vi "DMM Configuration - Update DMM Measurements ComboBox.vi"(8 "error in (no error)":errorcluster, 10 "Measurement":u16, 11 "Ring in":refnum<vi>) -> (0 "error out":errorcluster)   [LabVIEW 2015, in "DMM-SWITCH-ScanList System Explorer.lvlib"]
uses:
  DMM-SWITCH-ScanList System Explorer.lvlib
  Configuration Controls/DMM Config Function.ctl
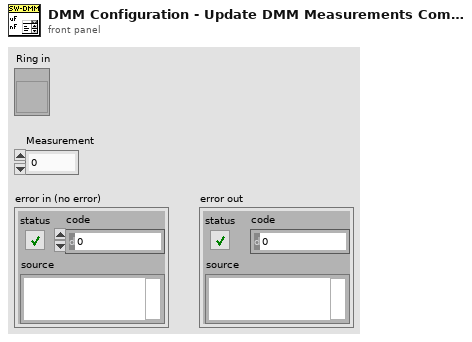
[diagram p1: front panel]
types:
  T1 = typedef "DMM-SWITCH-ScanList System Explorer.lvlib/DMM Config Function.ctl" = enum16{"DC Volts", "AC Volts", "DC Current", "AC Current", "2-wire Resistance", "4-wire Resistance", "Diode", "Frequency", "AC Volts DC Coupled", "Capacitance", "Inductance"}
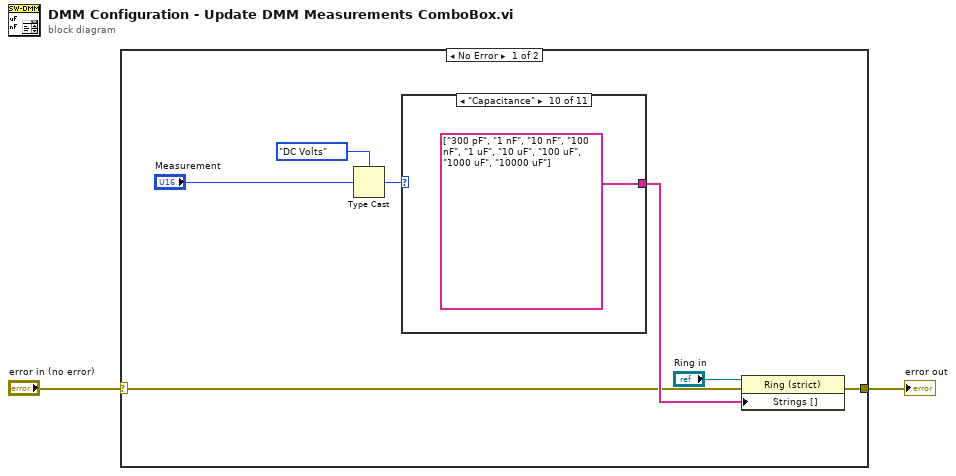
[diagram p0: block diagram]
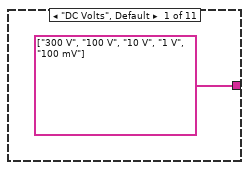
[diagram p2: hidden frame]
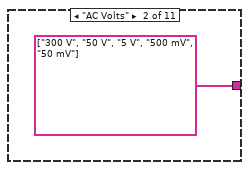
[diagram p3: hidden frame]
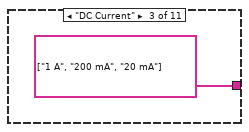
[diagram p4: hidden frame]
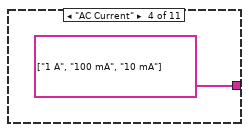
[diagram p5: hidden frame]
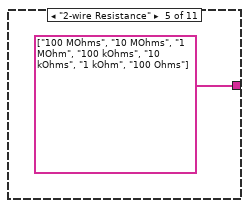
[diagram p6: hidden frame]
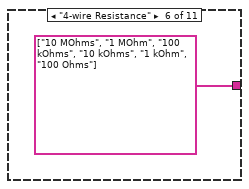
[diagram p7: hidden frame]
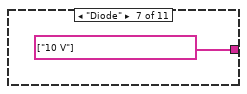
[diagram p8: hidden frame]
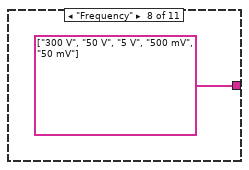
[diagram p9: hidden frame]
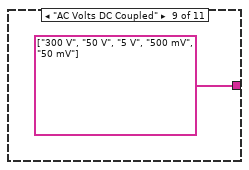
[diagram p10: hidden frame]
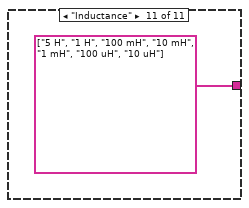
[diagram p11: hidden frame]
diagram:
  n1 = case shown="No Error" "error in (no error)" {
    selector: "error in (no error)" -> [w3 w21]
    tunnel: [w9 w21] -> w2
    frame No Error {
      n2 = Type Cast(type=DMM_Config_Function."DC Volts" ("Measurement Type Def"), x="Measurement") -> (*(type *) &x=w6:T1)
      n3 = case shown="\"Capacitance\"" w6 {
        tunnel: [string[] ["300 V", "100 V", "10 V", "1 V", "100 mV"] ("Strings []") string[] ["300 V", "50 V", "5 V", "500 mV", "50 mV"] ("Strings []") string[] ["1 A", "200 mA", "20 mA"] ("Strings []") string[] ["1 A", "100 mA", "10 mA"] ("Strings []") string[] ["100 MOhms", "10 MOhms", "1 MOhm", "100 kOhms", "10 kOhms", "1 kOhm", "100 Ohms"] ("Strings []") string[] ["10 MOhms", "1 MOhm", "100 kOhms", "10 kOhms", "1 kOhm", "100 Ohms"] ("Strings []") string[] ["10 V"] ("Strings []") string[] ["300 V", "50 V", "5 V", "500 mV", "50 mV"] ("Strings []") string[] ["300 V", "50 V", "5 V", "500 mV", "50 mV"] ("Strings []") string[] ["300 pF", "1 nF", "10 nF", "100 nF", "1 uF", "10 uF", "100 uF", "1000 uF", "10000 uF"] ("Strings []") string[] ["5 H", "1 H", "100 mH", "10 mH", "1 mH", "100 uH", "10 uH"] ("Strings []")] -> w5
        frame "DC Volts", Default {
        }
        frame "AC Volts" {
        }
        frame "DC Current" {
        }
        frame "AC Current" {
        }
        frame "2-wire Resistance" {
        }
        frame "4-wire Resistance" {
        }
        frame "Diode" {
        }
        frame "Frequency" {
        }
        frame "AC Volts DC Coupled" {
        }
        frame "Capacitance" {
        }
        frame "Inductance" {
        }
      }
      n4 = property on="Property Node" class="Ring (strict)"(reference="Ring in", error in=w3, "Strings []"=w5) -> (error out=w9:errorcluster)  [unwired: 1 out]
    }
    frame Error {
    }
  }
  "error out" <- w2
